vi "libssh2_userauth_list.vi"(8 "error in (no error)":errorcluster, 10 "username":string, 11 "session":u64) -> (0 "error out":errorcluster, 3 "return value":string)   [LabVIEW 2013, in "libssh2.lvlib"]
uses:
  libssh2.lvlib
  libssh2.dll
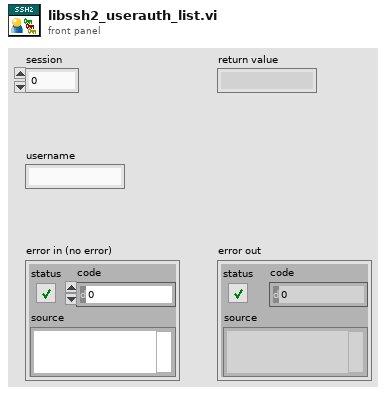
[diagram p1: front panel]
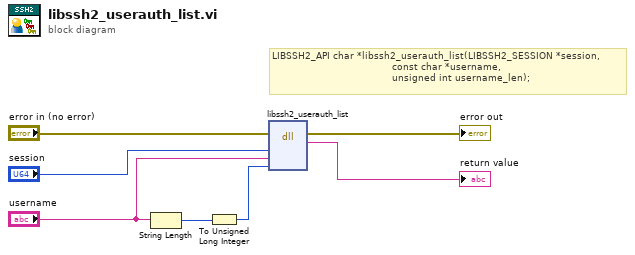
[diagram p0: block diagram]
diagram:
  # "LIBSSH2_API char *libssh2_userauth_list(LIBSSH2_SESSION *session,\n                                        const char *username,\n                                        unsigned int username_len);"
  n1 = String Length(string="username") -> (length=w1:i32)
  n2 = To Unsigned Long Integer(number=w1) -> (unsigned 32bit integer=w5:u32)
  n3 = dll-call lib="C:/Users/pasca/source/repos/libssh2-labview/libssh2**.*" fn="libssh2_userauth_list"(error in="error in (no error)", "session"="session", "username"="username", "username_len"=w5) -> (error out=→"error out":errorcluster, "return value"=→"return value":string)  [unwired: 5 in, 1 out]
